vi "Write Module Index.vi"(8 "error in (no error)":errorcluster, 10 "Module Index":u8, 11 "RemIO Module in":refnum<class "RemIO Module.lvclass">) -> (0 "error out":errorcluster, 3 "RemIO Module out":refnum<class "RemIO Module.lvclass">)   [LabVIEW 2016, in "Modules.lvlib" / "RemIO Module.lvclass"]
uses:
  RemIO Module.lvclass
  RemIO Module.lvclass/RemIO Module.ctl
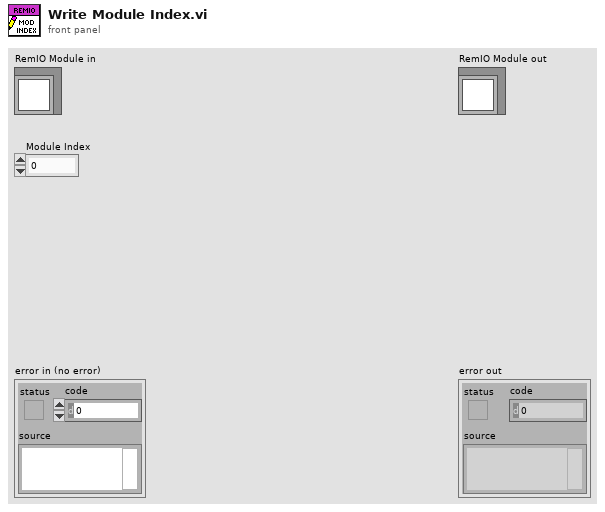
[diagram p1: front panel]
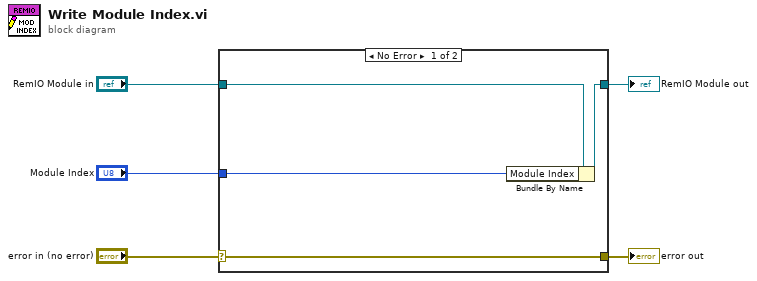
[diagram p0: block diagram]
diagram:
  n1 = case shown="No Error" "error in (no error)" {
    selector: "error in (no error)" -> [w9 w10]
    tunnel: [w9 w10] -> w4
    tunnel: [w7 w11] -> w2
    tunnel: "RemIO Module in" -> [w8 w11]
    tunnel: "Module Index" -> [w6 _]
    frame No Error {
      n2 = Bundle By Name(cluster=w8, "Module Index"=w6) -> (w7:refnum<class "RemIO Module.lvclass">)
    }
    frame Error {
    }
  }
  "error out" <- w4
  "RemIO Module out" <- w2
